vi "ЛР3 - 3 варик.vi"() -> ()   [LabVIEW 2012]
uses:
  <vilib>/express/express analysis/Spectral/Block/exnSpectralBlock spectral measurements power poly.vi
  <vilib>/express/express analysis/Spectral/Block/exnSpectralBlock spectral measurements power DDT.vi
  <vilib>/express/express analysis/Spectral/XNode/ExpressSpectralMeasurementsBlockNode.xnode
panel:
  out "Specific Harmonic":dbl
  out "THD":dbl
  in  "?":bool
  in  "Time Reg":dbl(slide) scale=500.0..2000.0
  out "Spectral":dynamicdata(graph)
  out "Arithmetic Mean":dbl
  out "Standard Dev":dbl
  out "Range":dbl
  out "Minimum":dbl
  in  "Bandpass":bool
  out "Maximum":dbl
  in  "Noise amplitude":dbl(slide)=0.6 scale=0.0..3.0
  out "Waveform Graph":dynamicdata(graph)
  in  "Amplitude":dbl(slide)=1.0 scale=0.0..10.0
  in  "Hz":dbl(knob)=10.1 caption="Frequency" scale=10.0..100.0
  # "Smothing"
  # "Filter"
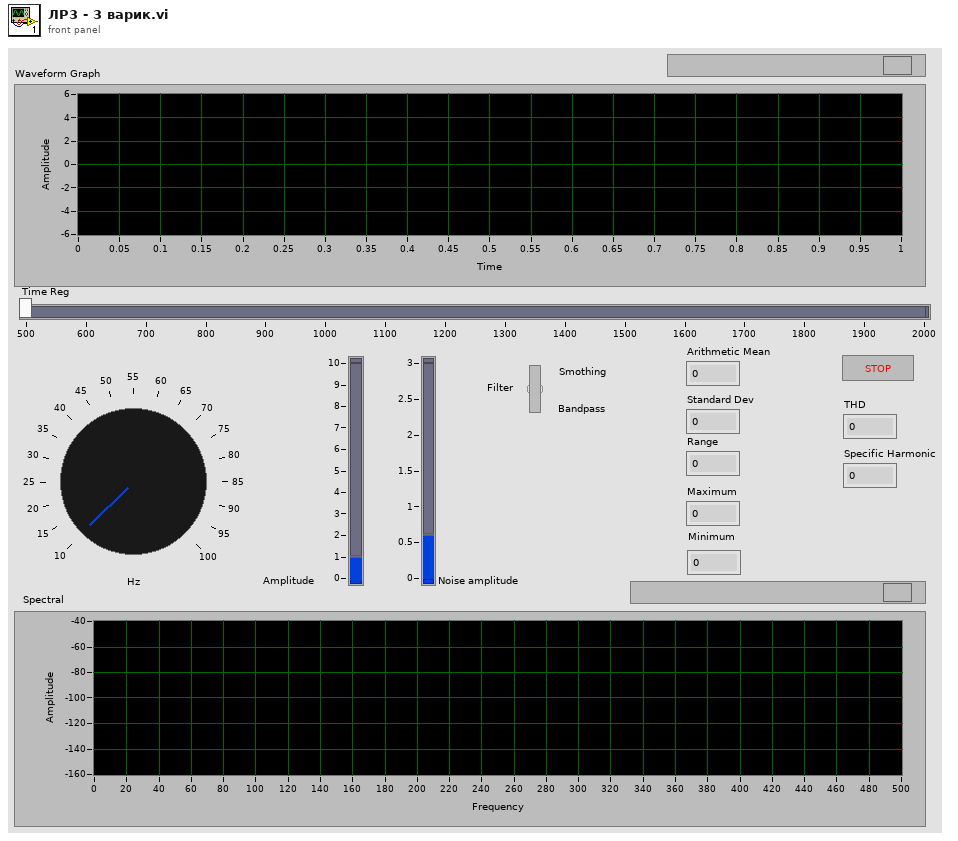
[diagram p1: front panel]
types:
  T1 = cluster{"averaging mode":u16, "weighting mode":u16, "number of averages":u32}
  T2 = cluster{"dB On (F)":bool, "unwrap phase (F)":bool, "convert to degree (F)":bool}
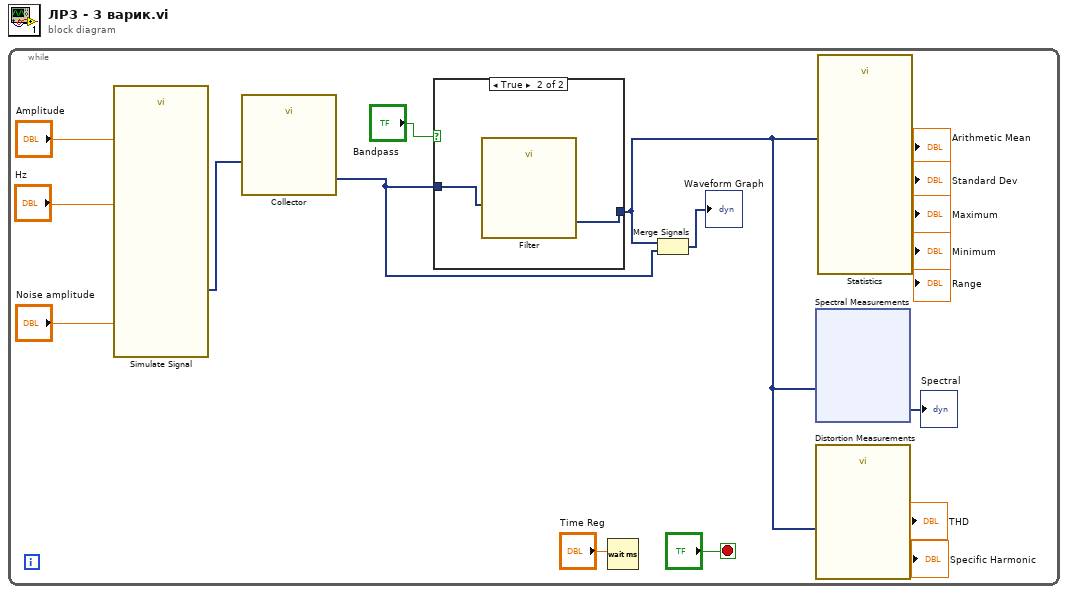
[diagram p0: block diagram]
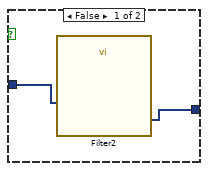
[diagram p2: hidden frame]
diagram:
  n1 = while {
    stop <- "?" stop-if-true
    n2 = call "Simulate Signal"("Frequency"="Hz", "Amplitude"="Amplitude", "Noise amplitude"="Noise amplitude") -> ("Sine with Uniform Noise"=w16:dynamicdata)  [unwired: 11 in, 1 out]
    n3 = call "Collector"("Signals"=w16) -> ("Collected Signals"=w15:dynamicdata)  [unwired: 9 in, 1 out]
    n4 = case shown="True" "Bandpass" {
      tunnel: w15 -> [w29 w31]
      tunnel: [w28 w30] -> w3
      frame False {
        n5 = call "Filter2"("Signal"=w29) -> ("Filtered Signal"=w28:dynamicdata)  [unwired: 9 in, 1 out]
      }
      frame True {
        n6 = call "Filter"("Signal"=w31) -> ("Filtered Signal"=w30:dynamicdata)  [unwired: 9 in, 1 out]
      }
    }
    n7 = Wait (ms)(milliseconds to wait="Time Reg") -> ()  [unwired: 1 out]
    n8 = Merge Signals(w3, w15) -> (→"Waveform Graph":dynamicdata)
    n9 = xnode "Spectral Measurements"("Signals"=w3) -> ("Power Spectrum"=→"Spectral":dynamicdata)  [unwired: 1 in, 1 out]
    n10 = call "Distortion Measurements"("Signals"=w3) -> ("Specific Harmonic"=→"Specific Harmonic":dynamicdata, "THD"=→"THD":dynamicdata)  [unwired: 8 in, 1 out]
    n11 = call "Statistics"("Signals"=w3) -> ("Standard Dev"=→"Standard Dev":dynamicdata, "Arithmetic Mean"=→"Arithmetic Mean":dynamicdata, "Range"=→"Range":dynamicdata, "Minimum"=→"Minimum":dynamicdata, "Maximum"=→"Maximum":dynamicdata)  [unwired: 21 in, 1 out]
  }
